vi "testerofmissionqueueadd.vi"() -> ()   [LabVIEW 2012]
uses:
  cRIO_Code/Data/TypeDefs/UTM Location.ctl
  cRIO_Code/Data/TypeDefs/MissionTypeControl.ctl
  cRIO_Code/Logic/Classes/Missions/GenericMission/GenericMission.lvclass
panel:
  out "queue out 2":refnum<queue>
  out "element":refnum<class "GenericMission.lvclass">
  in  "OK Button":bool
  in  "stop":bool
  out "queue out":refnum<queue>
  in  "Tolerance (m)":dbl
  in  "Timeout (s)":dbl=-1.0
  in  "Mission Type":T1
  in  "Duration (s)":dbl=-1.0
  in  "Error In":errorcluster
  in  "Points of Interest":T2[](array[typedef]) {"North" format="%#_10f"; "East" format="%#_8f"}
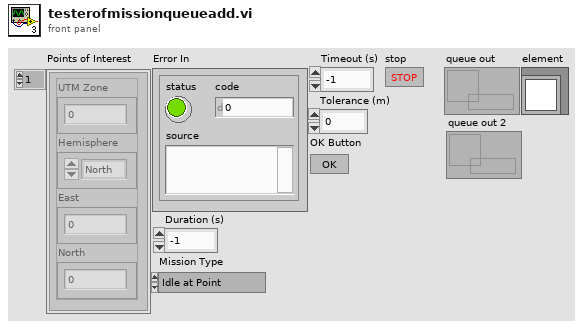
[diagram p1: front panel]
types:
  T1 = typedef "MissionTypeControl.ctl" = enum16{"Idle at Point", "Drive to Waypoint", "Round Buoy to Port", "Round Buoy to Starboard", "Pass Between Buoys", "Station Keeping"}
  T2 = typedef "UTM Location.ctl" = cluster{"UTM Zone":dbl, "Hemisphere":enum16{"North", "South"}, "East":dbl, "North":dbl}
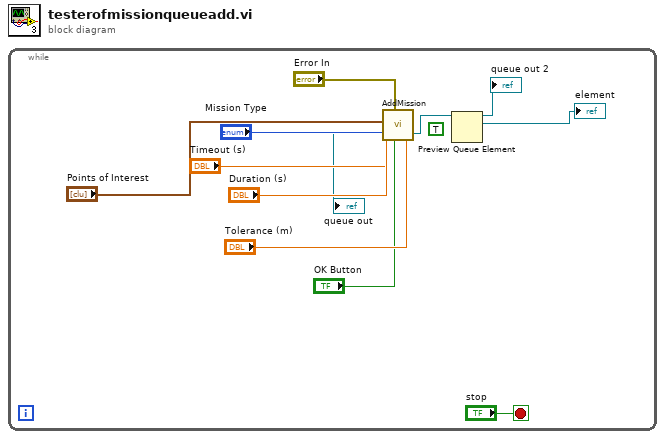
[diagram p0: block diagram]
diagram:
  n1 = while {
    stop <- "stop" stop-if-true
    (unwired) TRUE ("return elements? (F)")
    n2 = call "AddMission.vi"("Tolerance (m)"="Tolerance (m)", "OK Button"="OK Button", "Error In"="Error In", "Timeout (s)"="Timeout (s)", "Mission Type"="Mission Type", "Points of Interest"="Points of Interest", "Duration (s)"="Duration (s)") -> ("queue out"=w3:refnum<queue>)
    "queue out" <- w3
    n3 = Preview Queue Element(queue=w3) -> (queue out=→"queue out 2":refnum<queue>, element=→"element":refnum<class "GenericMission.lvclass">)  [unwired: 2 in, 2 out]
  }
